vi "Step4_inprogress.vi"() -> ()   [LabVIEW 2025]
uses:
  <vilib>/Utility/file.llb/Read Delimited Spreadsheet (DBL).vi
  <vilib>/express/express analysis/Spectral/Block/exnSpectralBlock spectral measurements peak poly.vi
  <vilib>/express/express analysis/Spectral/Block/exnSpectralBlock spectral measurements peak DDT.vi
  <vilib>/express/express analysis/Spectral/XNode/ExpressSpectralMeasurementsBlockNode.xnode
  <vilib>/Analysis/NI_AALBase.lvlib
  <vilib>/Analysis/NI_AAL_SigProc.lvlib
panel:
  out "Waveform Graph":dbl[](graph)
  out "Amplitudes":dbl[](array[numeric])
  out "Frequency":dbl[](array[numeric])
  out "Fourier Analysis":dynamicdata(graph)
  out "Filtered Signal":dynamicdata(graph)
  out "After Outlier Removal":waveform(dbl)(graph)
  in  "Z Threshold":dbl
  in  "Data File Path":path
  out "Time vs Signal":waveform(dbl)(graph)
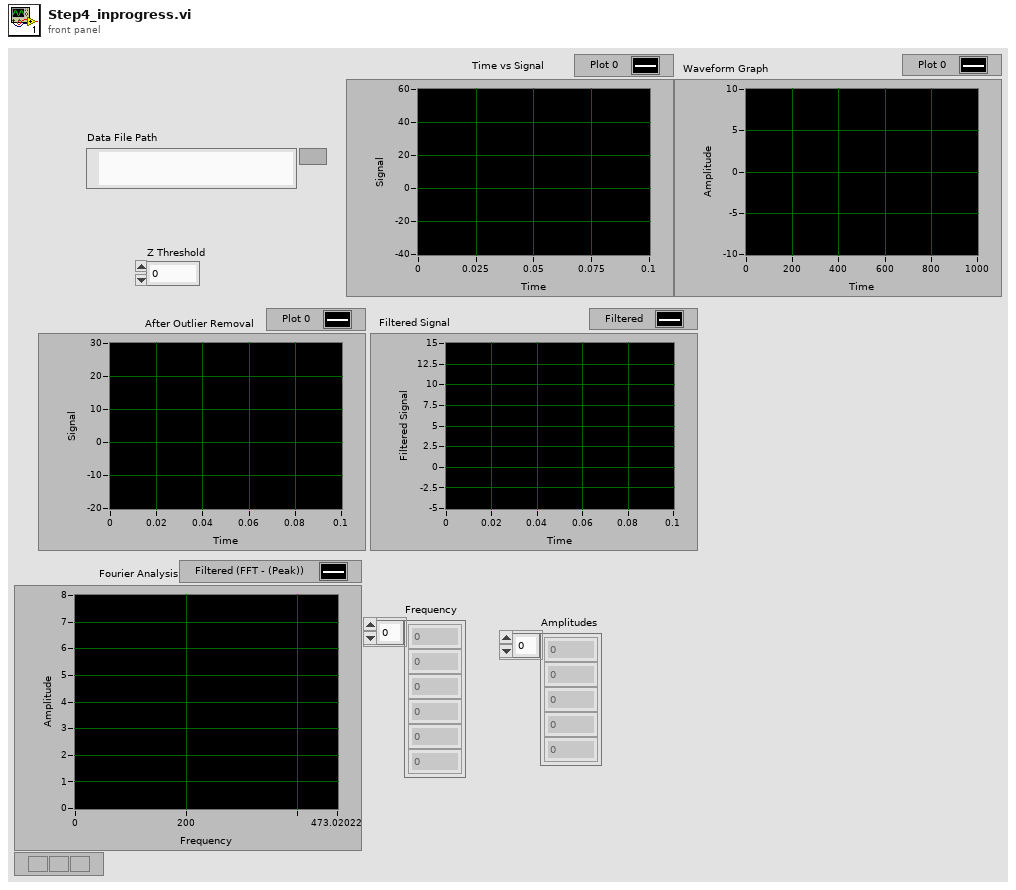
[diagram p1: front panel]
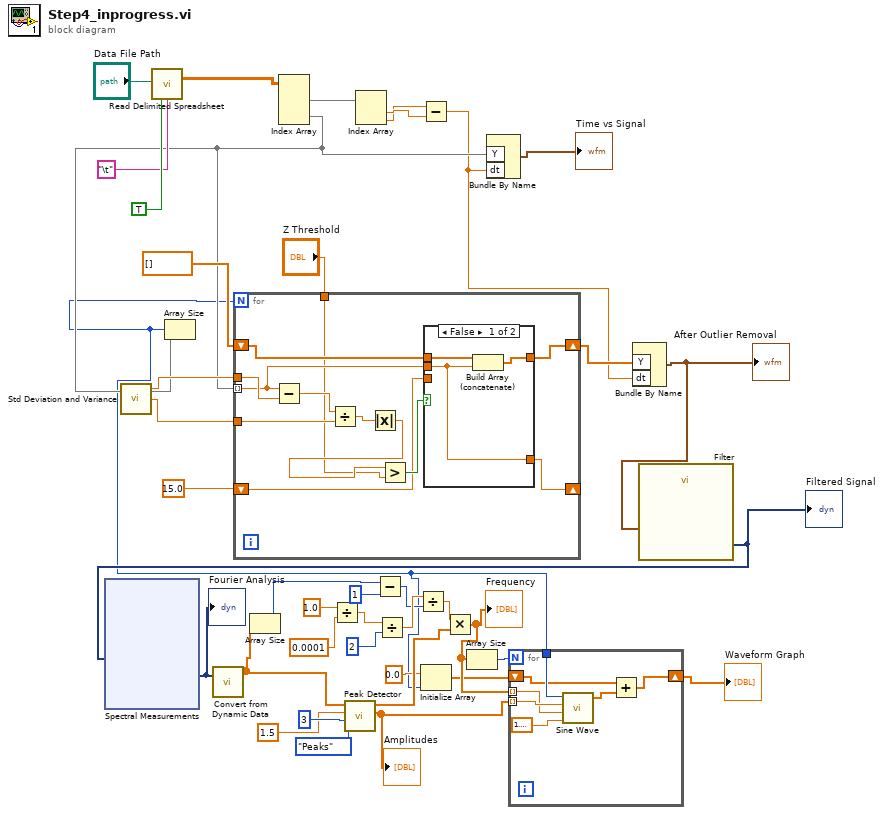
[diagram p0: block diagram]
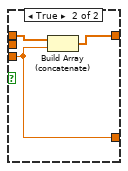
[diagram p2: hidden frame]
diagram:
  n1 = call-poly <vilib>:"Read Delimited Spreadsheet.vi"("file path (dialog if empty)"="Data File Path", "transpose? (F)"=TRUE, "delimiter (\\t)"="\t" ("delimiter (\\t)")) -> ("all rows"=w38:dbl[][])  [unwired: 7 in, 5 out]
  n2 = Index Array(array=w38) -> (element #1=w37:dbl[], element #2=w26:dbl[])  [unwired: 4 in]
  n3 = call <vilib>:"Std Deviation and Variance.vi"("X"=w26) -> ("mean"=w32:dbl, "standard deviation"=w31:dbl)  [unwired: 1 in, 1 out]
  n4 = Array Size(array=w26) -> (size(s)=w3:i32)
  n5 = for {
    N: w3 -> [_]
    shift-right: [w47] -> w28
    tunnel: w31 -> [w51]
    tunnel: w26 -> [w45] mode=indexing
    tunnel: w32 -> [w49]
    tunnel: "Z Threshold" -> [w41]
    shift-left: dbl[] [] -> [w46]
    shift-right: [w43] -> _
    shift-left: 15.0 -> [w44]
    n6 = Subtract(x=w45, y=w49) -> (x-y=w52:dbl)
    n7 = Divide(x=w52, y=w51) -> (x/y=w50:dbl)
    n8 = Absolute Value(x=w50) -> (abs(x)=w42:dbl)
    n9 = Greater?(x=w42, y=w41) -> (0:w48:bool)
    n10 = case shown="False" w48 {
      tunnel: w45 -> [w53 _]
      tunnel: w46 -> [w54 w58]
      tunnel: [w55 w57] -> w47
      tunnel: w44 -> [_ w56]
      tunnel: [w53 w56] -> w43
      frame False {
        n11 = Build Array (concatenate)(w54, w53) -> (w55:dbl[])
      }
      frame True {
        n12 = Build Array (concatenate)(w58, w56) -> (w57:dbl[])
      }
    }
  }
  n13 = Divide(x=1.0, y=0.0001) -> (x/y=w16:dbl)
  n14 = Index Array(array=w37) -> (element #1=w36:dbl, element #2=w27:dbl)  [unwired: 2 in]
  n15 = Divide(x=w16, y=2) -> (x/y=w14:dbl)
  n16 = Subtract(x=w27, y=w36) -> (x-y=w5:dbl)
  n17 = Initialize Array(0.0 ("element"), w3) -> (w2:dbl[])
  n18 = Bundle By Name("Y"=w26, "dt"=w5) -> (→"Time vs Signal":waveform(dbl))  [unwired: 1 in]
  n19 = Bundle By Name("Y"=w28, "dt"=w5) -> (w25:waveform(dbl))  [unwired: 1 in]
  "After Outlier Removal" <- w25
  n20 = call "Filter"("Signal"=w25) -> ("Filtered Signal"=w24:dynamicdata)  [unwired: 9 in, 1 out]
  "Filtered Signal" <- w24
  n21 = xnode "Spectral Measurements"("Signals"=w24) -> ("FFT - (Peak)"=w20:dynamicdata)  [unwired: 1 in, 2 out]
  "Fourier Analysis" <- w20
  n22 = call "Convert from Dynamic Data"("Dynamic Data Type"=w20) -> ("Array"=w19:dbl[])  [unwired: 3 in]
  n23 = Array Size(array=w19) -> (size(s)=w11:i32)
  n24 = call <vilib>:"Peak Detector.vi"("peaks/valleys"=enum32{"Peaks", "Valleys"}."Peaks", "width"=3, "threshold"=1.5, "X"=w19) -> ("Amplitudes"=w7:dbl[], "Locations"=w10:dbl[])  [unwired: 3 in, 3 out]
  "Amplitudes" <- w7
  n25 = Subtract(x=w11, y=1) -> (x-y=w13:i32)
  n26 = Divide(x=w14, y=w13) -> (x/y=w9:dbl)
  n27 = Multiply(x=w9, y=w10) -> (x*y=w6:dbl[])
  "Frequency" <- w6
  n28 = Array Size(array=w6) -> (size(s)=w8:i32)
  n29 = for {
    N: w8 -> [_]
    tunnel: w7 -> [w64] mode=indexing
    tunnel: w6 -> [w63] mode=indexing
    tunnel: w3 -> [w62]
    shift-right: [w59] -> w1
    shift-left: w2 -> [w60]
    n30 = call <vilib>:"Sine Wave.vi"("samples"=w62, "amplitude"=w64, "frequency"=w63, "phase in"=1.5707963267948966) -> ("sine wave"=w61:dbl[])  [unwired: 1 in, 2 out]
    n31 = Add(x=w60, y=w61) -> (x+y=w59:dbl[])
  }
  "Waveform Graph" <- w1
